vi "convert student data to boolean array.vi"(10 "Student data":i32[][](array[numeric])) -> (1 "expanded class data":bool[][](array[boolean]))   [LabVIEW 2009]
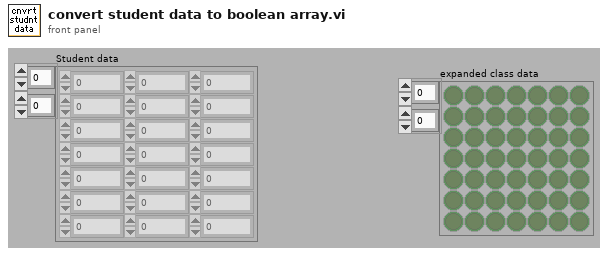
[diagram p1: front panel]
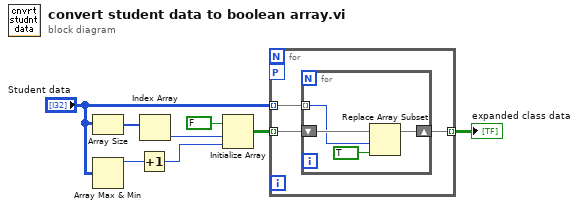
[diagram p0: block diagram]
diagram:
  n1 = Array Size(array="Student data") -> (size(s)=w3:i32[])
  n2 = Array Max & Min(array="Student data") -> (max value=w2:i32)  [unwired: 3 out]
  n3 = Increment(x=w2) -> (x+1=w5:i32)
  n4 = Index Array(array=w3) -> (element=w4:i32)  [unwired: 1 in]
  n5 = Initialize Array(FALSE, w4, w5) -> (w7:bool[][])
  n6 = for {
    tunnel: "Student data" -> [w11] mode=indexing
    tunnel: w7 -> [w10] mode=indexing
    tunnel: [w9] -> w8 mode=indexing
    workers-P: _ -> [_]
    n7 = for {
      tunnel: w11 -> [w14] mode=indexing
      shift-right: [w13] -> w9
      shift-left: w10 -> [w15]
      n8 = Replace Array Subset(array=w15, new element=TRUE ("new element/subarray"), index=w14) -> (w13:bool[])
    }
  }
  "expanded class data" <- w8
